vi "Cost.vi"(0 "reference in":refnum<class "Mocha.lvclass">, 5 "error in (no error)":errorcluster) -> (14 "reference out":refnum<class "Mocha.lvclass">, 16 "Cost($)":dbl, 19 "error out":errorcluster)   [LabVIEW 2020, in "Mocha.lvclass"]
uses:
  Mocha.lvclass
  C:/Projects/OpenGDS_DesignPatterns/Decorator1/CondimentDecorator_class/CondimentDecorator.lvclass
  Beverage_class/Beverage.lvclass
  CondimentDecorator_class/CondimentDecorator.lvclass
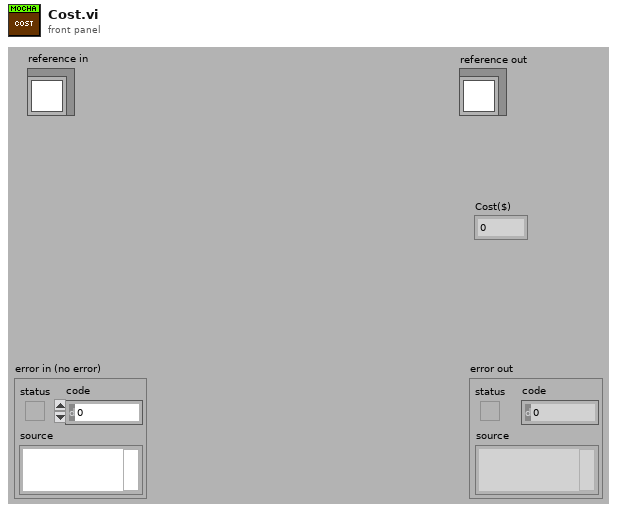
[diagram p1: front panel]
types:
  T1 = typedef "CondimentDecorator.lvclass/ObjectAttributes.ctl" = cluster{"BeverageRef":refnum<class "Beverage.lvclass">, "CondimentName":string}
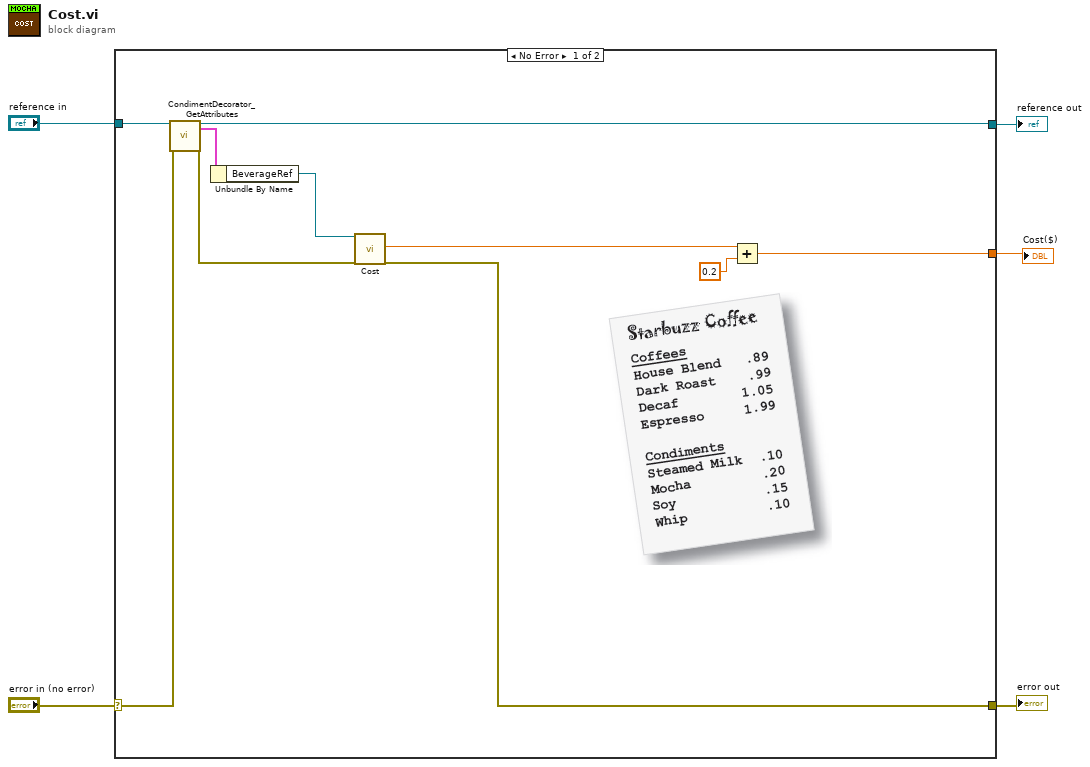
[diagram p0: block diagram]
diagram:
  n1 = case shown="No Error" "error in (no error)" {
    selector: "error in (no error)" -> [w14 w17]
    tunnel: [w6 w17] -> w4
    tunnel: [w13 w16] -> w2
    tunnel: "reference in" -> [w15 w16]
    tunnel: [w8 _] -> w1
    frame No Error {
      n2 = call "CondimentDecorator_GetAttributes.vi"("reference in"=w15, "error in (no error)"=w14) -> ("reference out"=w13:refnum<class "Mocha.lvclass">, "Data"=w12:T1, "error out"=w7:errorcluster)  [unwired: 14 in, 1 out]
      n3 = Unbundle By Name(w12) -> ("BeverageRef"=w11:refnum<class "Beverage.lvclass">)
      n4 = call-dynamic "Cost.vi"("reference in"=w11, "error in (no error)"=w7) -> ("Cost($)"=w10:dbl, "error out"=w6:errorcluster)  [unwired: 15 in, 1 out]
      n5 = Add(x=w10, y=0.2) -> (x+y=w8:dbl)
    }
    frame Error {
    }
  }
  "error out" <- w4
  "reference out" <- w2
  "Cost($)" <- w1
